vi "Write To Device.vi"(7 "Use Cached Data?":bool, 8 "Error In":errorcluster, 9 "Post Data":string="{\"target_change_pending\":true,\"target_temperature\":%0.1f}", 10 "Device Name":string, 11 "Nest Config":T1) -> (0 "Error Out":errorcluster, 3 "Nest Config":T1)   [LabVIEW 2013, in "LMH-Nest.lvlib"]
uses:
  LMH-Nest.lvlib
  Type Defs/Nest Config.ctl
  <vilib>/httpClient/ClientHandle.ctl
  Type Defs/Session Data.ctl
  Type Defs/Nest Error.ctl
  <vilib>/httpClient/POSTBuffer.vi
  <vilib>/httpClient/LabVIEWHTTPClient.lvlib
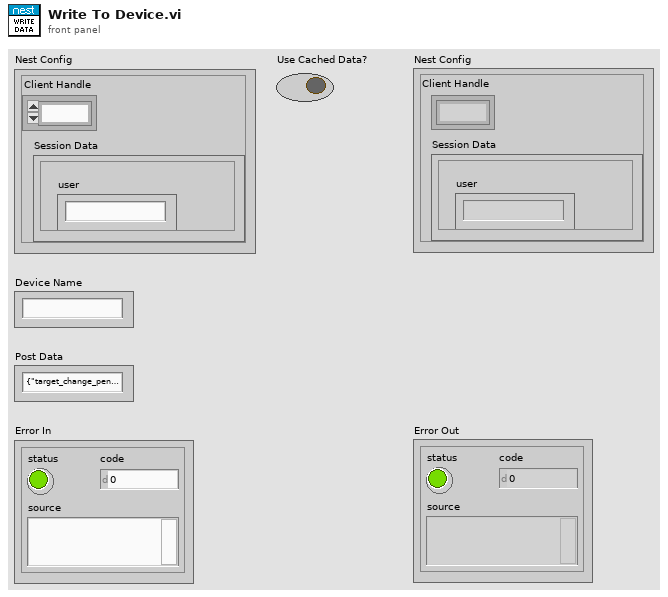
[diagram p1: front panel]
types:
  T1 = typedef "LMH-Nest.lvlib/Nest Config.ctl" = cluster{"Client Handle":T2, "Session Data":T3}
  T2 = typedef "LabVIEWHTTPClient.lvlib/ClientHandle.ctl" = refnum<k1>
  T3 = typedef "LMH-Nest.lvlib/Session Data.ctl" = cluster{"is_superuser":bool, "is_staff":bool, "urls":cluster{"transport_url":string, "rubyapi_url":string, "weather_url":string, "log_upload_url":string, "support_url":string}, "limits":cluster{"thermostats_per_structure":u32, "structures":u32, "thermostats":u32, "smoke_detectors":u32, "smoke_detectors_per_structure":u32}, "access_token":string, "userid":string, "expires_in":string, "email":string, "user":string, "language":string}
  T4 = typedef "LMH-Nest.lvlib/Nest Error.ctl" = enum16{"Unknown", "Auth", "Read", "Invalid Structure Name", "Invalid Device Name", "Set Temp"}
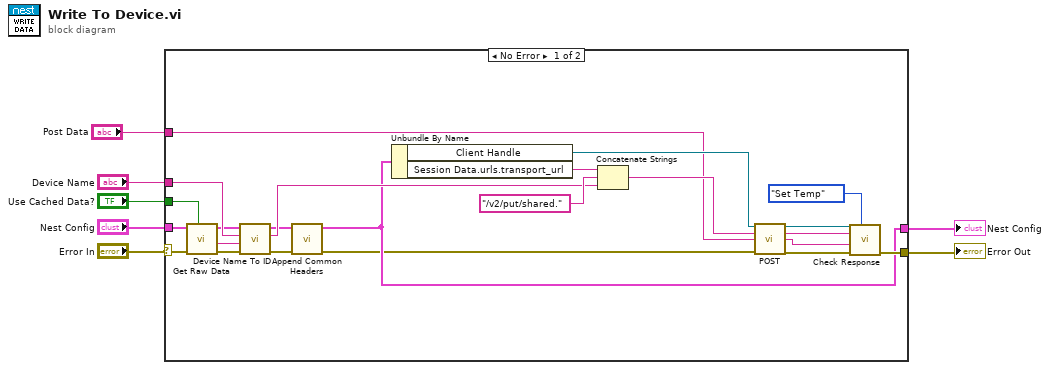
[diagram p0: block diagram]
diagram:
  n1 = case shown="No Error" "Error In" {
    selector: "Error In" -> [w28 w32]
    tunnel: "Use Cached Data?" -> [w30 _]
    tunnel: "Nest Config" -> [w29 w31]
    tunnel: "Device Name" -> [w25 _]
    tunnel: [w18 w32] -> w4
    tunnel: [w10 w31] -> w3
    tunnel: "Post Data" -> [w9 _]
    frame No Error {
      n2 = call "Get Raw Data.vi"("Use Cached Data?"=w30, "Error In"=w28, "Nest Config"=w29) -> ("Error Out"=w27:errorcluster, "Data"=w26:string, "Nest Config"=w24:T1)  [unwired: 6 in]
      n3 = call "Device Name To ID.vi"("Error In"=w27, "Data"=w26, "Device Name"=w25, "Nest Config"=w24) -> ("Error Out"=w12:errorcluster, "Device ID"=w22:string, "Nest Config"=w11:T1)  [unwired: 4 in, 1 out]
      n4 = call "Append Common Headers.vi"("Error In"=w12, "Nest Config"=w11) -> ("Error Out"=w8:errorcluster, "Nest Config"=w10:T1)  [unwired: 8 in]
      n5 = Unbundle By Name(w10) -> ("Client Handle"=w20:T2, "Session Data.urls.transport_url"=w21:string)
      n6 = Concatenate Strings(w21, "/v2/put/shared.", w22) -> (w19:string)
      n7 = call-poly <vilib>:"POST.vi"("client handle"=w20, "url"=w19, "buffer"=w9, "error in (no error)"=w8) -> ("client handle out"=w16:T2, "headers"=w14:string, "body"=w15:string, "error out"=w17:errorcluster)  [unwired: 8 in]
      n8 = call "Check Response.vi"("Nest Error"=Nest_Error."Set Temp", "Error In"=w17, "Body"=w15, "Header"=w14, "Client Handle"=w16) -> ("Error Out"=w18:errorcluster)  [unwired: 3 in, 3 out]
    }
    frame Error {
    }
  }
  "Error Out" <- w4
  "Nest Config" <- w3
